vi "Save TCP Msg.vi"(8 "error in (no error)":errorcluster, 11 "TCP Msg in":string) -> (0 "error out":errorcluster, 3 "TCP Msg out":string)   [LabVIEW 2019]
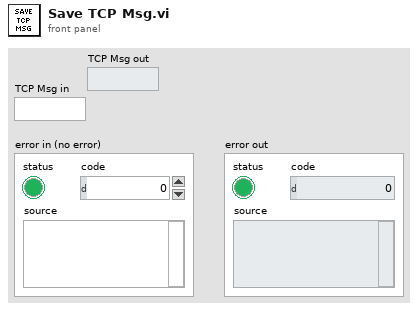
[diagram p1: front panel]
types:
  T1 = enum16{"open", "replace", "create", "open or create", "replace or create", "replace or create with confirmation"}
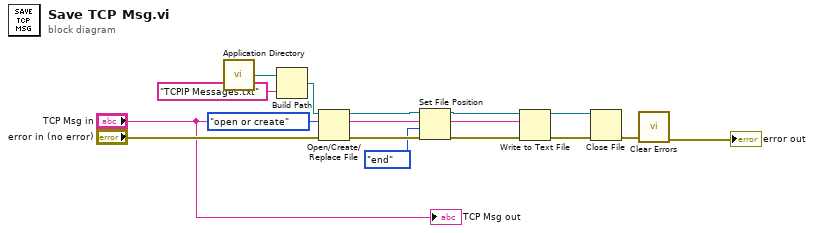
[diagram p0: block diagram]
diagram:
  n1 = call <vilib>:"Application Directory.vi"() -> ("Application Directory"=w8:path)
  n2 = Build Path(base path=w8, name or relative path="TCPIP Messages.txt") -> (appended path=w10:path)
  n3 = Open/Create/Replace File(file path (use dialog)=w10, error in="error in (no error)", operation (0:open)=T1."open or create") -> (refnum out=w5:refnum<file>, error out=w3:errorcluster)  [unwired: 3 in, 1 out]
  n4 = Set File Position(refnum=w5, from (0:start)=enum16{"start", "end", "current"}."end", error in=w3) -> (refnum out=w4:refnum<file>, error out=w2:errorcluster)  [unwired: 1 in]
  n5 = Write to Text File(file (use dialog)=w4, text="TCP Msg in", error in=w2) -> (refnum out=w12:refnum<file>, error out=w11:errorcluster)  [unwired: 1 in, 1 out]
  n6 = Close File(refnum=w12, error in=w11) -> (error out=w13:errorcluster)  [unwired: 1 out]
  n7 = call <vilib>:"Clear Errors.vi"("error in (no error)"=w13) -> ("error out"=→"error out":errorcluster)  [unwired: 5 in, 1 out]
  "TCP Msg out" <- "TCP Msg in"
